vi "Execute GC Helium Test.vi"(8 "error in":errorcluster, 9 "Test Results":T1, 10 "Gas":T3, 11 "GC Configuration":T4) -> (0 "error out":errorcluster, 1 "Test Results Out":T1, 2 "Gas Out":T3 caption="Gas", 3 "GC Configuration Out":T4)   [LabVIEW 2015]
uses:
  Controls/Test Information.ctl
  Controls/Vacuum Test.ctl
  Controls/Test Timing.ctl
  Controls/Vaccum Thresholds.ctl
  Controls/Helium Test.ctl
  Controls/Helium Thresholds.ctl
  CAN Communication/Gas/Typedefs/Session Handle.ctl
  CAN Communication/Gas/Gas.lvclass
  Controls/Test Results.ctl
  Controls/Step Result.ctl
  User Interface/UI Handler/UI Handler.lvclass
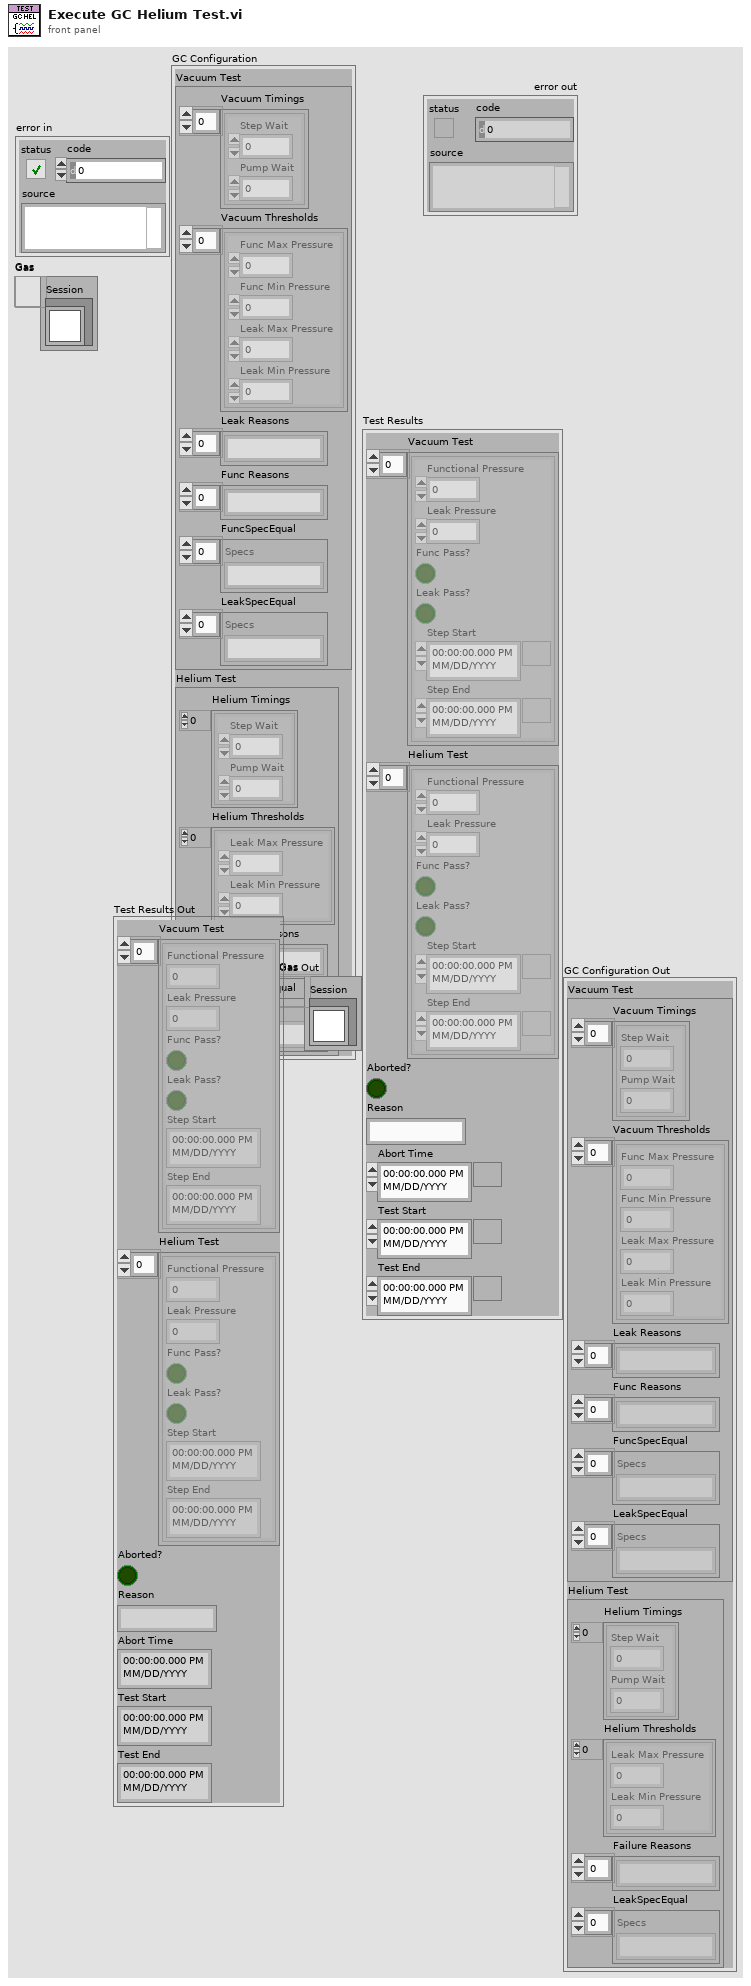
[diagram p1: front panel]
types:
  T1 = typedef "Test Results.ctl" = cluster{"Vacuum Test":T2[], "Helium Test":T2[], "Aborted?":bool, "Reason":string, "Abort Time":timestamp, "Test Start":timestamp, "Test End":timestamp}
  T2 = typedef "Step Result.ctl" = cluster{"Functional Pressure":dbl, "Leak Pressure":dbl, "Func Pass?":bool, "Leak Pass?":bool, "Step Start":timestamp, "Step End":timestamp}
  T3 = typedef "Gas.lvclass/Session Handle.ctl" = refnum<data-value>
  T4 = typedef "Test Information.ctl" = cluster{"Vacuum Test":T5, "Helium Test":T8}
  T5 = typedef "Vacuum Test.ctl" = cluster{"Vacuum Timings":T6[], "Vacuum Thresholds":T7[], "Leak Reasons":string[], "Func Reasons":string[], "FuncSpecEqual":string[], "LeakSpecEqual":string[]}
  T6 = typedef "Test Timing.ctl" = cluster{"Step Wait":dbl, "Pump Wait":dbl}
  T7 = typedef "Vaccum Thresholds.ctl" = cluster{"Func Max Pressure":dbl, "Func Min Pressure":dbl, "Leak Max Pressure":dbl, "Leak Min Pressure":dbl}
  T8 = typedef "Helium Test.ctl" = cluster{"Helium Timings":T6[], "Helium Thresholds":T9[], "Failure Reasons":string[], "LeakSpecEqual":string[]}
  T9 = typedef "Helium Thresholds.ctl" = cluster{"Leak Max Pressure":dbl, "Leak Min Pressure":dbl}
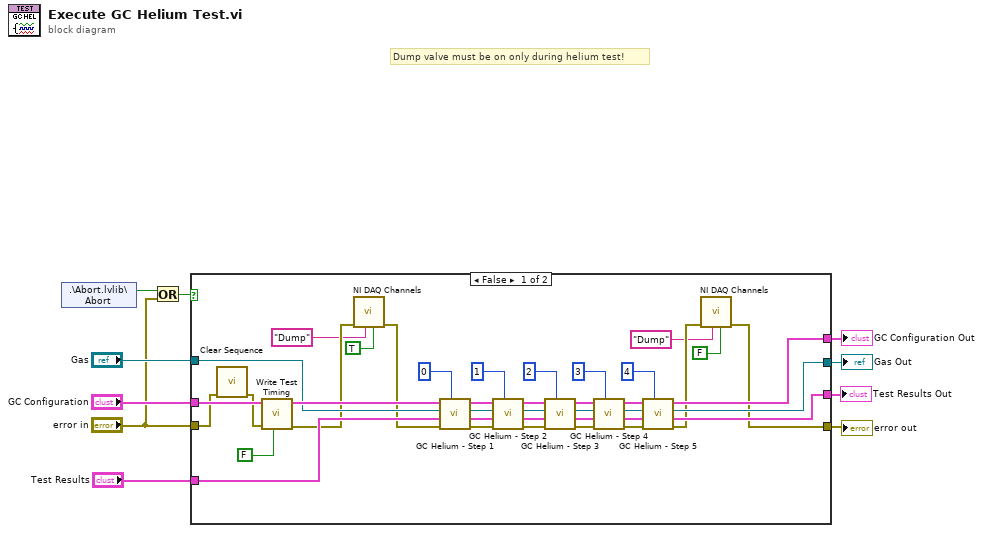
[diagram p0: block diagram]
diagram:
  # "Dump valve must be on only during helium test!"
  n1 = shared-variable ".\\Abort.lvlib\\Abort"() -> (w3:bool)  [unwired: 1 in, 1 out]
  n2 = Or(x=w3, y="error in") -> (x .or. y?=w2:bool)
  n3 = case shown="False" w2 {
    tunnel: "error in" -> [w20 w49]
    tunnel: "GC Configuration" -> [w47 w52]
    tunnel: "Gas" -> [w46 w51]
    tunnel: "Test Results" -> [w45 w50]
    tunnel: [w23 w52] -> w7
    tunnel: [w22 w51] -> w6
    tunnel: [w21 w50] -> w5
    tunnel: [w13 w49] -> w4
    frame False {
      n4 = call "Clear Sequence.vi"("error in (no error)"=w20) -> ("error out"=w19:errorcluster)  [unwired: 10 in]
      n5 = call "Write Test Timing.vi"("Vacuum?"=FALSE, "error in (no error)"=w19, "Test Information"=w47) -> ("error out"=w18:errorcluster)  [unwired: 8 in]
      n6 = call "NI DAQ Channels.vi"("Control"=TRUE, "Channel"="Dump", "error in (no error)"=w18) -> ("error out"=w17:errorcluster)  [unwired: 7 in, 1 out]
      n7 = call "GC Helium - Step 1.vi"("Step"=0, "error in"=w17, "Test Results In"=w45, "Gas"=w46, "GC Configuration"=w47) -> ("error out"=w40:errorcluster, "Test Results Out"=w41:T1, "Gas Out"=w42:T3, "GC Configuration Out"=w43:T4)  [unwired: 3 in]
      n8 = call "GC Helium - Step 2.vi"("Step"=1, "error in"=w40, "Test Results In"=w41, "Gas"=w42, "GC Configuration"=w43) -> ("error out"=w38:errorcluster, "Test Results Out"=w35:T1, "Gas Out"=w36:T3, "GC Configuration Out"=w37:T4)  [unwired: 3 in]
      n9 = call "GC Helium - Step 3.vi"("Step"=2, "error in"=w38, "Test Results In"=w35, "Gas"=w36, "GC Configuration"=w37) -> ("error out"=w33:errorcluster, "Test Results Out"=w30:T1, "Gas Out"=w31:T3, "GC Configuration Out"=w32:T4)  [unwired: 3 in]
      n10 = call "GC Helium - Step 4.vi"("Step"=3, "error in"=w33, "Test Results In"=w30, "Gas"=w31, "GC Configuration"=w32) -> ("error out"=w27:errorcluster, "Test Results Out"=w25:T1, "Gas Out"=w26:T3, "GC Configuration Out"=w28:T4)  [unwired: 3 in]
      n11 = call "GC Helium - Step 5.vi"("Step"=4, "error in"=w27, "Test Results In"=w25, "Gas"=w26, "GC Configuration"=w28) -> ("error out"=w14:errorcluster, "Test Results Out"=w21:T1, "Gas Out"=w22:T3, "GC Configuration Out"=w23:T4)  [unwired: 3 in]
      n12 = call "NI DAQ Channels.vi"("Control"=FALSE, "Channel"="Dump", "error in (no error)"=w14) -> ("error out"=w13:errorcluster)  [unwired: 7 in, 1 out]
    }
    frame True {
    }
  }
  "error out" <- w4
  "GC Configuration Out" <- w7
  "Gas Out" <- w6
  "Test Results Out" <- w5
